vi "自定义插值.vi"(9 "压力":dbl, 10 "压力数组":dbl[](array[numeric]), 11 "扭矩数组":dbl[](array[numeric])) -> (2 "扭矩值":dbl)   [LabVIEW 2011]
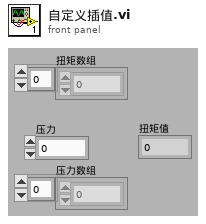
[diagram p1: front panel]
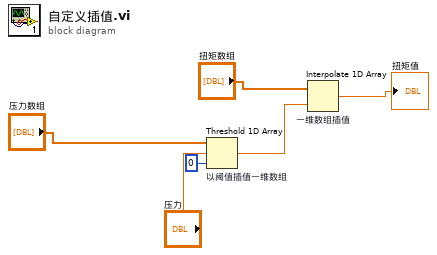
[diagram p0: block diagram]
diagram:
  n1 = Threshold 1D Array "以阈值插值一维数组"(1:0 ("开始索引(0)"), 2:"压力", 3:"压力数组") -> (0:w5:dbl)
  n2 = Interpolate 1D Array "一维数组插值"(1:w5, 2:"扭矩数组") -> (0:→"扭矩值":dbl)
